vi "ContourPlot multi-channel v1.5.vi"() -> ()   [LabVIEW 2024]
uses:
  <vilib>/Utility/file.llb/Read Delimited Spreadsheet (DBL).vi
  <vilib>/gmath/NI_Gmath.lvlib
  <vilib>/Analysis/NI_AALPro.lvlib
panel:
  out "Channel number":i32=2
  out "Ready?":bool=TRUE
  in  "Tab Control 2":enum32{"Contour"}(tab)
  out "Intensity Graph":dbl[][](graph)
  in  "Begin":i32
  in  "x label index":i32
  in  "y label index":i32=1
  in  "intensisty plot channel index":i32
  in  "y cut x index":i32=1
  in  "length":i32=200
  out "Y cut plot":cluster{dbl[], "Best Polynomial Fit":dbl[]}[](graph)=[{[0.01650390625, 0.02626953125, 0.03503417969, 0.05258789063, 0.06340332031, 0.0546875, 0.07456054687, 0.08317871094, 0.08818359375, 0.09924316406, 0.1127685547, 0.1196777344, 0.1380615234, 0.1424804688, 0.148046875, 0.1650146484, 0.1830322266, 0.1841552734, 0.1907714844, 0.2046386719, 0.2173339844, 0.2219238281, 0.2336425781, 0.2451171875, 0.2626464844, 0.2627197266, 0.2696044922, 0.2876708984, 0.2832763672, 0.2978027344, 0.3136474609, 0.3143798828, 0.3297607422, 0.3401123047, 0.3473144531, 0.355859375, 0.3647460938, 0.3720703125, 0.3781738281, 0.3934082031, 0.4053955078, 0.4169189453, 0.4156494141, 0.4353027344, 0.4502685547, 0.4522949219, 0.4749755859, 0.4762451172, 0.4824707031, 0.4980957031, 0.5044433594, 0.5147216797, 0.5253662109, 0.5385253906, 0.552734375, 0.5608886719, 0.5664306641, 0.5922607422, 0.5865966797, 0.5947509766, 0.6063476562, 0.6142089844, 0.6204345703, 0.6424804687, 0.6439697266, 0.6533691406, 0.6609863281, 0.6897460937, 0.6840820313, 0.7033203125, 0.7142822266, 0.7231201172, 0.7217285156, 0.7270019531, 0.7446777344, 0.7530273438, 0.7546875, 0.7791503906, 0.7783203125, 0.8080810547, 0.8064208984, 0.8069335937, 0.8181640625, 0.8277099609, 0.8401367187, 0.8624023438, 0.8599365234, 0.8799316406, 0.8899169922, 0.8873779297, 0.9, 0.9150390625, 0.9197753906, 0.9276367187, 0.93984375, 0.9463378906, 0.9627929687, 0.9658447266, 0.9845458984, 0.9911865234, 1.010253906, 1.012182617, 1.013989258, 1.03515625, 1.044555664, 1.054956055, 1.057836914, 1.068212891, 1.084838867, 1.094091797, 1.110571289, 1.110839844, 1.119702148, 1.134082031, 1.137158203, 1.161303711, 1.157958984, 1.169970703, 1.183227539, 1.180249023, 1.200537109, 1.208227539, 1.218481445, 1.234399414, 1.243554688, 1.252514648, 1.253100586, 1.276611328, 1.281152344, 1.289453125, 1.303710937, 1.309399414, 1.324316406, 1.327954102, 1.337182617, 1.351611328, 1.34831543, 1.378686523, 1.3796875, 1.387011719, 1.411791992, 1.400170898, 1.414160156, 1.420532227, 1.436669922, 1.440698242, 1.455786133, 1.459790039, 1.479541016, 1.489038086, 1.496142578, 1.511181641, 1.512011719, 1.534008789, 1.534716797, 1.537475586, 1.548364258, 1.570654297, 1.579516602, 1.589624023, 1.589770508, 1.612304687, 1.609423828, 1.624584961, 1.635961914, 1.650219727, 1.652270508, 1.659472656, 1.675244141, 1.690478516, 1.698364258, 1.712353516, 1.714160156, 1.720214844, 1.747485352, 1.749584961, 1.757861328, 1.76862793, 1.776074219, 1.789038086, 1.783422852, 1.798583984, 1.815722656, 1.82565918, 1.828222656, 1.847949219, 1.852368164, 1.857226562, 1.877050781, 1.876049805, 1.894042969, 1.902758789, 1.906469727, 1.93112793, 1.926000977, 1.941088867, 1.946313477, 1.962207031, 1.96887207, 1.978833008], "Best Polynomial Fit"=[2.522949219e-05, 2.175537109e-05, 2.422851563e-05, 2.607177734e-05, 2.364990234e-05, 2.185546875e-05, 2.321044922e-05, 2.395507813e-05, 2.384277344e-05, 2.321289062e-05, 2.442382813e-05, 2.266357422e-05, 2.279052734e-05, 2.379150391e-05, 2.479248047e-05, 2.408935547e-05, 2.789306641e-05, 2.418701172e-05, 2.358154297e-05, 2.761962891e-05, 2.335205078e-05, 2.244384766e-05, 2.471191406e-05, 2.399414063e-05, 2.87890625e-05, 2.490234375e-05, 2.447265625e-05, 2.583496094e-05, 2.252929688e-05, 2.367919922e-05, 2.464111328e-05, 2.297363281e-05, 2.394287109e-05, 2.505371094e-05, 2.201904297e-05, 2.275878906e-05, 2.444824219e-05, 2.458496094e-05, 2.179931641e-05, 2.502685547e-05, 2.063964844e-05, 2.412353516e-05, 2.250976563e-05, 2.124755859e-05, 2.354003906e-05, 2.381835938e-05, 2.278320313e-05, 2.311767578e-05, 2.487548828e-05, 2.473632813e-05, 2.686767578e-05, 2.40234375e-05, 2.554931641e-05, 2.405273438e-05, 2.608398438e-05, 2.446533203e-05, 2.228027344e-05, 2.522705078e-05, 2.221923828e-05, 2.467041016e-05, 2.422851563e-05, 2.247314453e-05, 2.319580078e-05, 2.590332031e-05, 2.395263672e-05, 2.550292969e-05, 2.307617188e-05, 2.522216797e-05, 2.477783203e-05, 2.593261719e-05, 2.587890625e-05, 2.457519531e-05, 2.587646484e-05, 2.187988281e-05, 2.429443359e-05, 2.553222656e-05, 2.353271484e-05, 2.535400391e-05, 2.636474609e-05, 2.397949219e-05, 2.451904297e-05, 2.4453125e-05, 2.314208984e-05, 2.224121094e-05, 2.318847656e-05, 2.693603516e-05, 2.556152344e-05, 2.429443359e-05, 2.602539063e-05, 2.283935547e-05, 2.181640625e-05, 2.506591797e-05, 2.462890625e-05, 2.314941406e-05, 2.465332031e-05, 2.322753906e-05, 2.138671875e-05, 2.248779297e-05, 2.436523437e-05, 2.090576172e-05, 2.705566406e-05, 2.369384766e-05, 2.477783203e-05, 2.453125e-05, 2.129150391e-05, 2.686523438e-05, 2.388671875e-05, 2.263671875e-05, 2.577636719e-05, 2.232421875e-05, 2.777099609e-05, 2.622070313e-05, 2.127441406e-05, 2.596923828e-05, 2.402099609e-05, 2.520263672e-05, 2.533691406e-05, 2.317138672e-05, 2.414550781e-05, 2.462646484e-05, 2.55859375e-05, 2.456054688e-05, 2.296630859e-05, 2.576416016e-05, 2.376220703e-05, 2.401123047e-05, 2.224121094e-05, 2.405029297e-05, 2.700683594e-05, 2.282958984e-05, 2.713867187e-05, 2.715820313e-05, 2.547851562e-05, 2.447265625e-05, 2.329345703e-05, 2.407714844e-05, 1.942382813e-05, 2.3828125e-05, 2.417236328e-05, 2.610107422e-05, 2.278808594e-05, 2.241943359e-05, 2.251220703e-05, 2.4609375e-05, 2.484619141e-05, 2.555908203e-05, 2.657714844e-05, 2.638427734e-05, 2.3515625e-05, 2.619140625e-05, 2.568603516e-05, 2.450683594e-05, 2.463134766e-05, 2.594482422e-05, 2.453125e-05, 2.508056641e-05, 2.398193359e-05, 2.307373047e-05, 2.713867187e-05, 2.829589844e-05, 2.318847656e-05, 2.735839844e-05, 2.381591797e-05, 2.542236328e-05, 2.177001953e-05, 2.354492187e-05, 2.625976563e-05, 2.388427734e-05, 2.348876953e-05, 2.697509766e-05, 2.808837891e-05, 2.255371094e-05, 2.540771484e-05, 2.225097656e-05, 2.594482422e-05, 2.569824219e-05, 2.602539063e-05, 2.532470703e-05, 2.746582031e-05, 2.675537109e-05, 2.2109375e-05, 2.42578125e-05, 2.152587891e-05, 2.559082031e-05, 2.332275391e-05, 2.565917969e-05, 2.493164063e-05, 2.20703125e-05, 2.518798828e-05, 2.071289062e-05, 2.197753906e-05, 2.547851562e-05, 2.424316406e-05, 2.627685547e-05, 2.090576172e-05, 2.405273438e-05, 2.386962891e-05, 2.246826172e-05, 2.632568359e-05, 2.224853516e-05]}, {[0.01650390625, 0.02626953125, 0.03503417969, 0.05258789063, 0.06340332031, 0.0546875, 0.07456054687, 0.08317871094, 0.08818359375, 0.09924316406, 0.1127685547, 0.1196777344, 0.1380615234, 0.1424804688, 0.148046875, 0.1650146484, 0.1830322266, 0.1841552734, 0.1907714844, 0.2046386719, 0.2173339844, 0.2219238281, 0.2336425781, 0.2451171875, 0.2626464844, 0.2627197266, 0.2696044922, 0.2876708984, 0.2832763672, 0.2978027344, 0.3136474609, 0.3143798828, 0.3297607422, 0.3401123047, 0.3473144531, 0.355859375, 0.3647460938, 0.3720703125, 0.3781738281, 0.3934082031, 0.4053955078, 0.4169189453, 0.4156494141, 0.4353027344, 0.4502685547, 0.4522949219, 0.4749755859, 0.4762451172, 0.4824707031, 0.4980957031, 0.5044433594, 0.5147216797, 0.5253662109, 0.5385253906, 0.552734375, 0.5608886719, 0.5664306641, 0.5922607422, 0.5865966797, 0.5947509766, 0.6063476562, 0.6142089844, 0.6204345703, 0.6424804687, 0.6439697266, 0.6533691406, 0.6609863281, 0.6897460937, 0.6840820313, 0.7033203125, 0.7142822266, 0.7231201172, 0.7217285156, 0.7270019531, 0.7446777344, 0.7530273438, 0.7546875, 0.7791503906, 0.7783203125, 0.8080810547, 0.8064208984, 0.8069335937, 0.8181640625, 0.8277099609, 0.8401367187, 0.8624023438, 0.8599365234, 0.8799316406, 0.8899169922, 0.8873779297, 0.9, 0.9150390625, 0.9197753906, 0.9276367187, 0.93984375, 0.9463378906, 0.9627929687, 0.9658447266, 0.9845458984, 0.9911865234, 1.010253906, 1.012182617, 1.013989258, 1.03515625, 1.044555664, 1.054956055, 1.057836914, 1.068212891, 1.084838867, 1.094091797, 1.110571289, 1.110839844, 1.119702148, 1.134082031, 1.137158203, 1.161303711, 1.157958984, 1.169970703, 1.183227539, 1.180249023, 1.200537109, 1.208227539, 1.218481445, 1.234399414, 1.243554688, 1.252514648, 1.253100586, 1.276611328, 1.281152344, 1.289453125, 1.303710937, 1.309399414, 1.324316406, 1.327954102, 1.337182617, 1.351611328, 1.34831543, 1.378686523, 1.3796875, 1.387011719, 1.411791992, 1.400170898, 1.414160156, 1.420532227, 1.436669922, 1.440698242, 1.455786133, 1.459790039, 1.479541016, 1.489038086, 1.496142578, 1.511181641, 1.512011719, 1.534008789, 1.534716797, 1.537475586, 1.548364258, 1.570654297, 1.579516602, 1.589624023, 1.589770508, 1.612304687, 1.609423828, 1.624584961, 1.635961914, 1.650219727, 1.652270508, 1.659472656, 1.675244141, 1.690478516, 1.698364258, 1.712353516, 1.714160156, 1.720214844, 1.747485352, 1.749584961, 1.757861328, 1.76862793, 1.776074219, 1.789038086, 1.783422852, 1.798583984, 1.815722656, 1.82565918, 1.828222656, 1.847949219, 1.852368164, 1.857226562, 1.877050781, 1.876049805, 1.894042969, 1.902758789, 1.906469727, 1.93112793, 1.926000977, 1.941088867, 1.946313477, 1.962207031, 1.96887207, 1.978833008], "Best Polynomial Fit"=[2.3228795830769698e-05, 2.341069346366108e-05, 2.355504147991162e-05, 2.3795519405393273e-05, 2.391469906466257e-05, 2.3820284520124616e-05, 2.401710940979356e-05, 2.4083254900352232e-05, 2.4116888297857293e-05, 2.417975023043444e-05, 2.4237284543491398e-05, 2.4259359660405112e-05, 2.4297365678530806e-05, 2.4302527066994272e-05, 2.430709334103077e-05, 2.4309247635142932e-05, 2.4295677584275923e-05, 2.4294390212520876e-05, 2.4285909030414153e-05, 2.426382232743864e-05, 2.423961165989159e-05, 2.4230148911820358e-05, 2.420474498304174e-05, 2.4178702256432762e-05, 2.413809533096356e-05, 2.413792586502446e-05, 2.4122068153247183e-05, 2.408168103479258e-05, 2.409128550544006e-05, 2.40602426719594e-05, 2.4029119842078877e-05, 2.4027762001171274e-05, 2.4001098745241157e-05, 2.3985289969419927e-05, 2.397537631628508e-05, 2.3964815474921127e-05, 2.3955252565574683e-05, 2.3948480492373423e-05, 2.3943611224214343e-05, 2.3934543789892576e-05, 2.3930494557852824e-05, 2.392912165406224e-05, 2.3929153642764616e-05, 2.393187743218695e-05, 2.393838559748473e-05, 2.3939546312950203e-05, 2.3956771526783283e-05, 2.395795320393103e-05, 2.396405879861498e-05, 2.398151997155728e-05, 2.3989416308291107e-05, 2.4003083872694712e-05, 2.4018271882353802e-05, 2.4038295012871163e-05, 2.4061174823473107e-05, 2.407476876491032e-05, 2.4084159409718046e-05, 2.4128931093897265e-05, 2.41190275799789e-05, 2.413328980614232e-05, 2.4153566159679614e-05, 2.4167231707166706e-05, 2.417796918245362e-05, 2.4215020315544587e-05, 2.421745211179008e-05, 2.423254227494948e-05, 2.4244410577196353e-05, 2.4285688461349103e-05, 2.4278049031381684e-05, 2.4302899628806453e-05, 2.4315592542593103e-05, 2.432499282953925e-05, 2.4323563432301958e-05, 2.432887805523345e-05, 2.4344617917373366e-05, 2.4350907330139375e-05, 2.435206831810665e-05, 2.4365672797342782e-05, 2.4365319581297557e-05, 2.4373213772416386e-05, 2.4373030356769133e-05, 2.4373090207897526e-05, 2.4373686013241878e-05, 2.437313154100677e-05, 2.4370988412561934e-05, 2.436332218384911e-05, 2.436440251089335e-05, 2.4354091150244176e-05, 2.4347690402125148e-05, 2.4349392119753666e-05, 2.434045956135379e-05, 2.4328383364058924e-05, 2.4324291850239552e-05, 2.4317228719890078e-05, 2.4305664413195e-05, 2.4299258201429508e-05, 2.428241499949932e-05, 2.427921642558946e-05, 2.425932582847943e-05, 2.4252212647697625e-05, 2.423196470857647e-05, 2.4229947905135855e-05, 2.4228066279712132e-05, 2.420674559521028e-05, 2.4197845486520096e-05, 2.4188529572252444e-05, 2.4186060654904753e-05, 2.417761630593956e-05, 2.4165736425936328e-05, 2.4160124404331738e-05, 2.4152134496050522e-05, 2.4152027020219336e-05, 2.414891409834052e-05, 2.4145743602599573e-05, 2.4145382808585117e-05, 2.414670574140505e-05, 2.4146067668272524e-05, 2.4149067848212727e-05, 2.4154711883147672e-05, 2.4153226041524322e-05, 2.4165904392509487e-05, 2.4172301617286524e-05, 2.4182216867140978e-05, 2.4200773527796116e-05, 2.4213194961081926e-05, 2.4226583300545907e-05, 2.422750108308381e-05, 2.426854401857523e-05, 2.4277402670570564e-05, 2.429435248766385e-05, 2.432568249131472e-05, 2.4338935906559334e-05, 2.43756213479775e-05, 2.438497239609259e-05, 2.4409364854176795e-05, 2.444929351301051e-05, 2.443999157466549e-05, 2.4529188288595783e-05, 2.453224475064365e-05, 2.455478945062161e-05, 2.463284879451093e-05, 2.459596878044354e-05, 2.4640402371289317e-05, 2.4660763431228958e-05, 2.471233820351259e-05, 2.472515816108467e-05, 2.4772706505834033e-05, 2.478515092076746e-05, 2.4844946786404913e-05, 2.4872482402446116e-05, 2.4892434513846227e-05, 2.4932519173232696e-05, 2.4934637143129816e-05, 2.4986565721917507e-05, 2.4988090871464093e-05, 2.4993939060424103e-05, 2.5015484577399667e-05, 2.50511256715321e-05, 2.5061787335741575e-05, 2.5071280314922957e-05, 2.5071396200998866e-05, 2.508139487184327e-05, 2.508101249043288e-05, 2.5079922617728644e-05, 2.5073917651267062e-05, 2.505981775529839e-05, 2.5057172194115074e-05, 2.5046627692103945e-05, 2.5016614432057417e-05, 2.4978446776763308e-05, 2.495511868258471e-05, 2.4907754575233254e-05, 2.49010838615088e-05, 2.48778136920395e-05, 2.47560482008859e-05, 2.4745568453862603e-05, 2.4702809288685255e-05, 2.4643877542225925e-05, 2.4601077615185943e-05, 2.452297323226292e-05, 2.455733152968015e-05, 2.4462904462535517e-05, 2.4350806303571892e-05, 2.4284071694797085e-05, 2.426672944834396e-05, 2.4132952886881873e-05, 2.41032171235233e-05, 2.4070775940738046e-05, 2.3943019980762065e-05, 2.394922994445811e-05, 2.384325159577108e-05, 2.3797238139455085e-05, 2.3778955372403057e-05, 2.368256158719051e-05, 2.3698512282108175e-05, 2.3658913078691834e-05, 2.365078435756507e-05, 2.3646900161595e-05, 2.365578698321734e-05, 2.3682270055891408e-05]}]
  out "Contour":cluster{dbl[], "Intensity Graph":dbl[]}(graph)={[-1.0, -0.9, -0.8, -0.7, -0.6, -0.5, -0.4, -0.3, -0.2, -0.1, 0.0, 0.1, 0.2, 0.3, 0.4, 0.5, 0.6], "Intensity Graph"=[5100.604889456126, -2470.3463533267786, -634.7944754974578, 10094.369029377345, -5260.545329369828, -207591.59935302305, -1145597.900176921, 501993.89566245984, -411866.74052445486, -492657.58824001026, 1411148.0553569798, 1597.6662420338712, -6432.561102017044, 6389.987173062791, -7753.278633121495, 3521.5036972613993, -2067.527503347544]}
  in  "threshold":dbl=0.18 step=0.01
  in  "extract method":string(combo)="Raw Data"
  in  "book number":i32=786
  in  "file path (dialog if empty)":path=path "C:/Users/gyue/Desktop/20221209 G22L measurement"
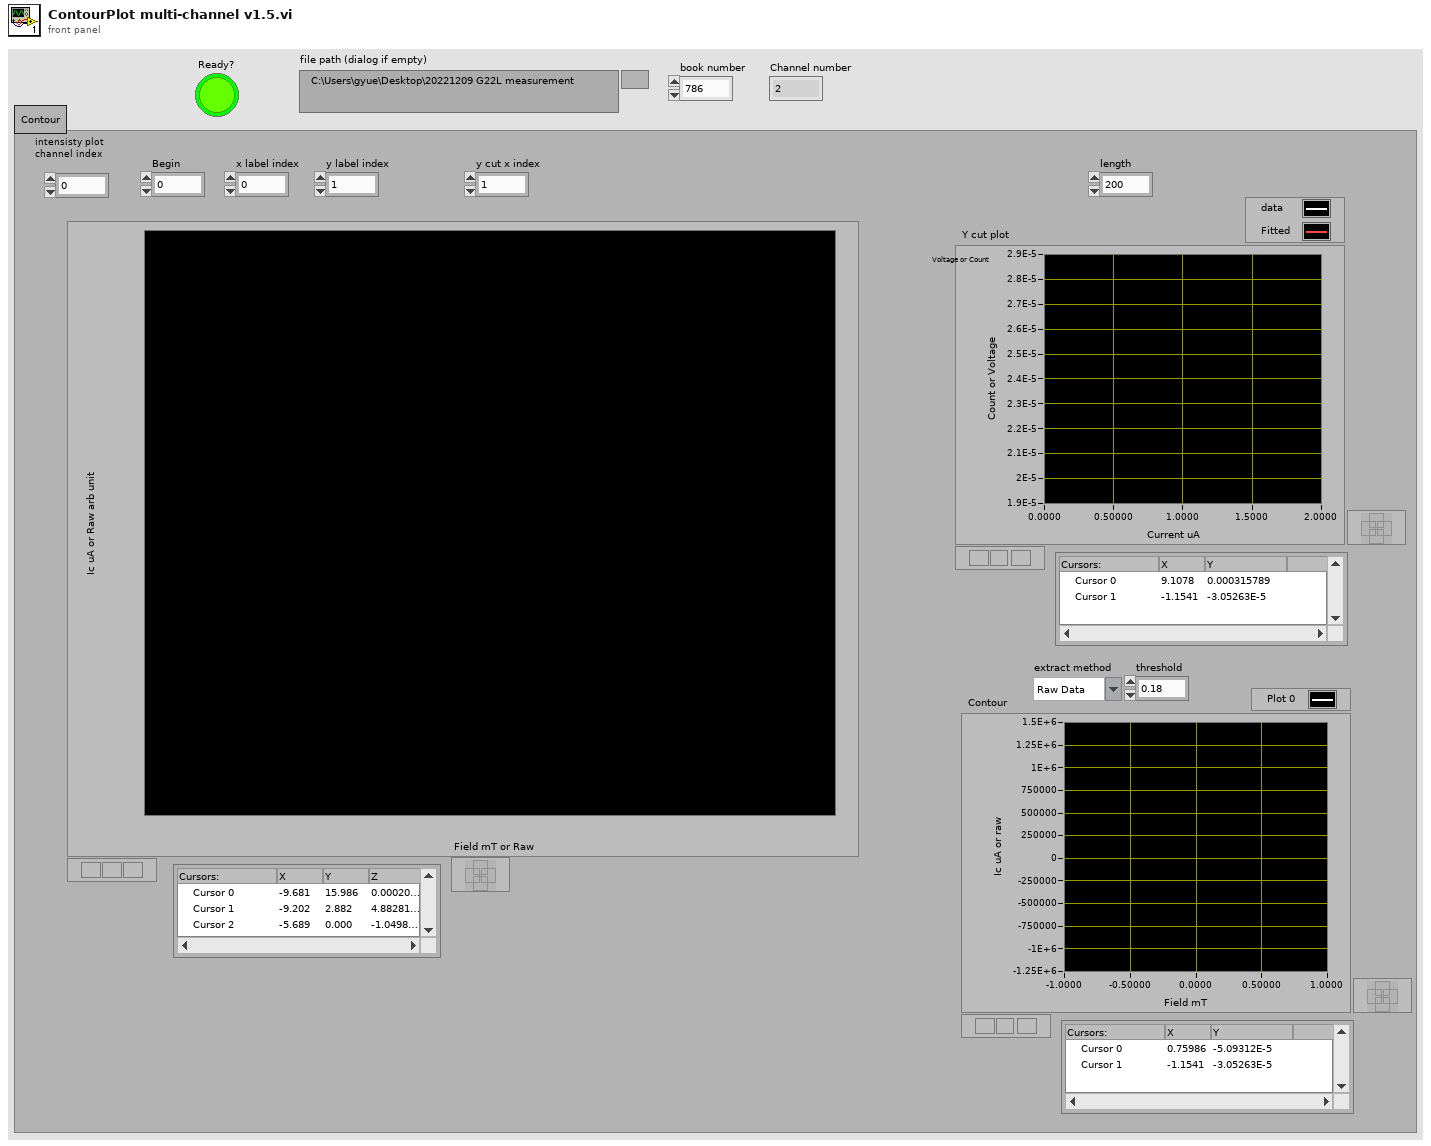
[diagram p1: front panel]
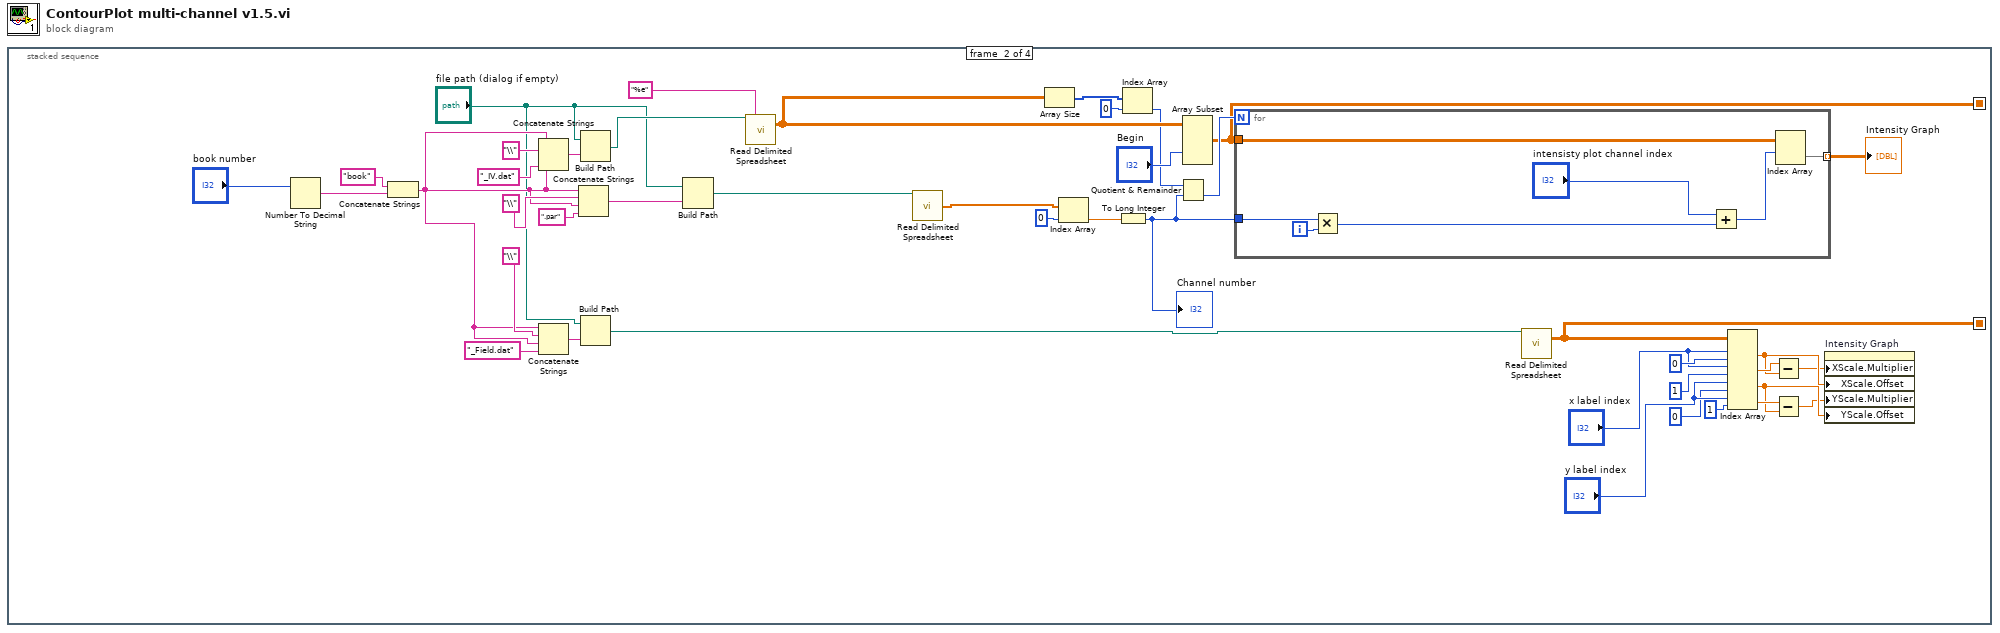
[diagram p0: block diagram]
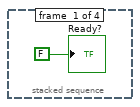
[diagram p2: hidden frame]
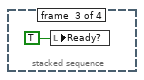
[diagram p3: hidden frame]
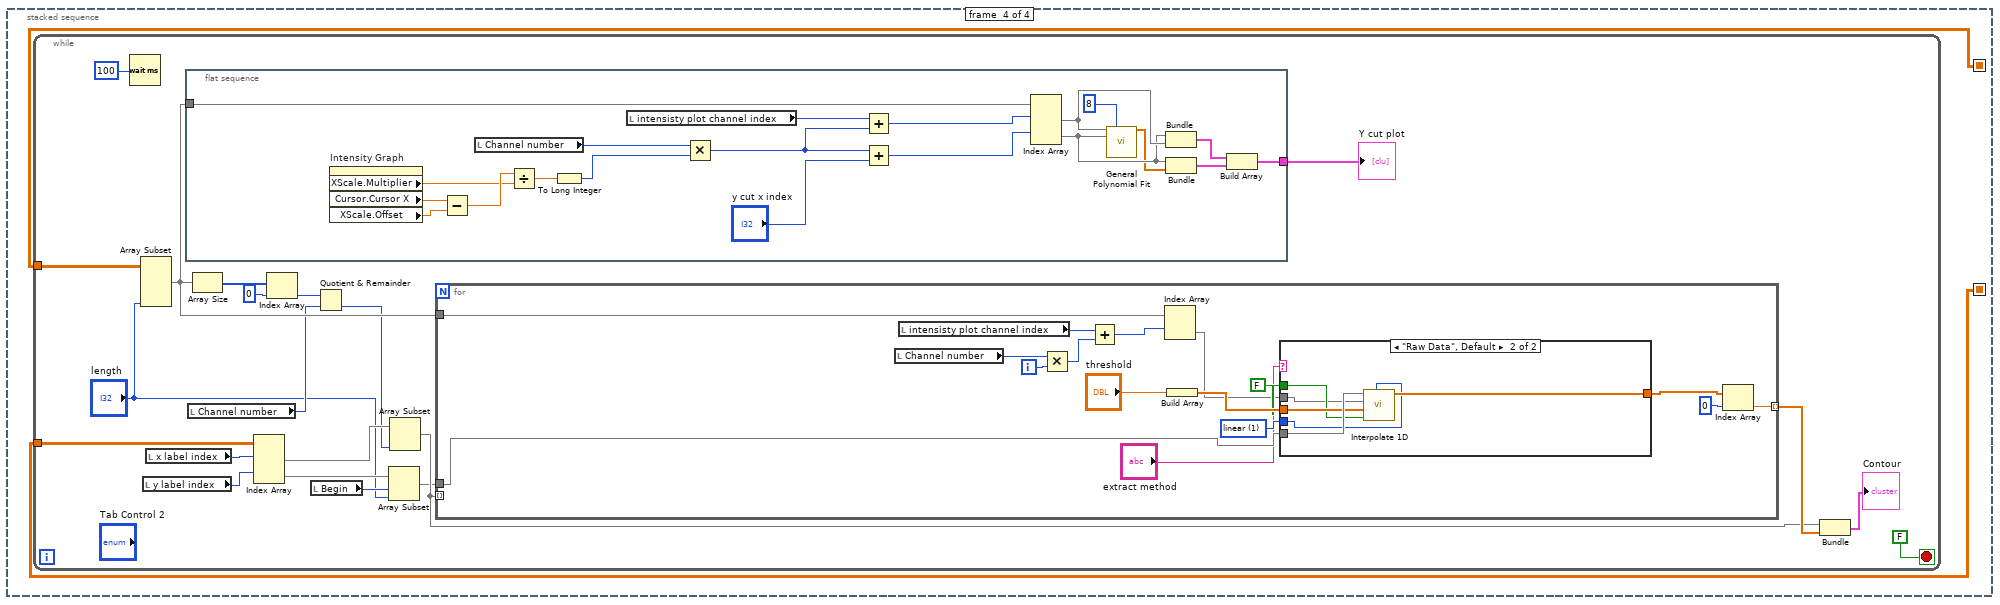
[diagram p4: hidden frame]
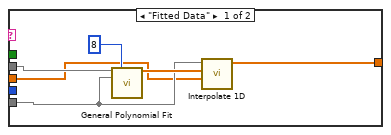
[diagram p5: hidden frame]
diagram:
  n1 = stacked-sequence {
    seq-local: [_ w3 _ _] -> [_ _ _ w53]
    seq-local: [_ w2 _ _] -> [_ _ _ w54]
    frame #0 {
      "Ready?" <- FALSE ("Ready?")
    }
    frame #1 {
      n2 = Number To Decimal String(number="book number") -> (decimal integer string=w40:string)  [unwired: 1 in]
      n3 = Concatenate Strings("book" ("string"), w40) -> (w29:string)
      n4 = Concatenate Strings(w29, "\\" ("string"), w29, "_IV.dat" ("string")) -> (w41:string)
      n5 = Concatenate Strings(w29, "\\" ("string"), w29, "_Field.dat" ("string")) -> (w23:string)
      n6 = Concatenate Strings(w29, "\\" ("string"), w29, ".par" ("string")) -> (w42:string)
      n7 = Build Path(base path="file path (dialog if empty)", name or relative path=w41) -> (appended path=w44:path)
      n8 = Build Path(base path="file path (dialog if empty)", name or relative path=w23) -> (appended path=w16:path)
      n9 = Build Path(base path="file path (dialog if empty)", name or relative path=w42) -> (appended path=w43:path)
      n10 = call-poly <vilib>:"Read Delimited Spreadsheet.vi"("file path (dialog if empty)"=w44, "format (%.3f)"="%e") -> ("all rows"=w26:dbl[][])  [unwired: 8 in, 5 out]
      n11 = call-poly <vilib>:"Read Delimited Spreadsheet.vi"("file path (dialog if empty)"=w43) -> ("first row"=w22:dbl[])  [unwired: 9 in, 5 out]
      n12 = Array Size(array=w26) -> (size(s)=w34:i32[])
      n13 = Index Array(array=w22, index=0) -> (element=w20:dbl)
      n14 = To Long Integer(number=w20) -> (32bit integer=w18:i32)
      "Channel number" <- w18
      n15 = Index Array(array=w34, index=0) -> (element=w19:i32)
      n16 = Quotient & Remainder(x=w19, y=w18) -> (floor(x/y)=w17:i32)  [unwired: 1 out]
      n17 = Array Subset(array=w26, index (col)="Begin") -> (w3:dbl[][])  [unwired: 3 in]
      n18 = for {
        N: w17 -> [_]
        tunnel: w3 -> [w50]
        tunnel: [w49] -> w27 mode=indexing
        tunnel: w18 -> [w46]
        i -> [w51]
        n19 = Multiply(x=w46, y=w51) -> (x*y=w45:i32)
        n20 = Add(x="intensisty plot channel index", y=w45) -> (x+y=w48:i32)
        n21 = Index Array(array=w50, index (row)=w48) -> (element=w49:dbl[])  [unwired: 1 in]
      }
      "Intensity Graph" <- w27
      n22 = call-poly <vilib>:"Read Delimited Spreadsheet.vi"("file path (dialog if empty)"=w16) -> ("all rows"=w2:dbl[][])  [unwired: 9 in, 5 out]
      n23 = Index Array(array=w2, index (row) #1="x label index", index (col) #1=0 ("disabled index (col)"), index (row) #2="x label index", index (col) #2=1 ("disabled index (col)"), index (row) #3="y label index", index (col) #3=0 ("disabled index (col)"), index (row) #4="y label index", index (col) #4=1 ("disabled index (col)")) -> (element #1=w11:dbl, element #2=w12:dbl, element #3=w5:dbl, element #4=w6:dbl)
      n24 = Subtract(x=w12, y=w11) -> (x-y=w10:dbl)
      n25 = Subtract(x=w6, y=w5) -> (x-y=w4:dbl)
      n26 = property on="Intensity Graph" class="IntGraph (strict)"("XScale.Multiplier"=w10, "XScale.Offset"=w11, "YScale.Multiplier"=w4, "YScale.Offset"=w5) -> ()  [unwired: 2 in, 2 out]
    }
    frame #2 {
      n27 = local write "Ready?"(TRUE ("Ready?")) -> ()
    }
    frame #3 {
      n28 = while {
        tunnel: w54 -> [w68]
        tunnel: w53 -> [w67]
        stop <- FALSE stop-if-true
        n29 = Wait (ms)(milliseconds to wait=u32 100) -> ()  [unwired: 1 out]
        n30 = Array Subset(array=w67, length (col)="length") -> (w66:dbl[][])  [unwired: 3 in]
        n31 = local read "y label index"() -> (w70:i32)
        n32 = local read "x label index"() -> (w69:i32)
        n33 = flat-sequence {
          tunnel: [w104] -> w75
          tunnel: w66 -> [w118]
          frame #0 {
            n34 = property on="Intensity Graph" class="IntGraph (strict)"() -> ("XScale.Multiplier"=w122:dbl, "Cursor.Cursor X"=w121:dbl, "XScale.Offset"=w120:dbl)  [unwired: 2 in, 2 out]
            n35 = Subtract(x=w121, y=w120) -> (x-y=w123:dbl)
            n36 = local read "Channel number"() -> (w116:i32)
            n37 = Divide(x=w123, y=w122) -> (x/y=w119:dbl)
            n38 = To Long Integer(number=w119) -> (32bit integer=w117:i32)
            n39 = local read "intensisty plot channel index"() -> (w114:i32)
            n40 = Multiply(x=w116, y=w117) -> (x*y=w115:i32)
            n41 = Add(x=w114, y=w115) -> (x+y=w113:i32)
            n42 = Add(x=w115, y="y cut x index") -> (x+y=w112:i32)
            n43 = Index Array(array=w118, index (row) #1=w113, index (row) #2=w112) -> (element #1=w110:dbl[], element #2=w108:dbl[])  [unwired: 2 in]
            n44 = call <vilib>:"General Polynomial Fit.vi"("Y"=w110, "polynomial order"=8, "X"=w108) -> ("Best Polynomial Fit"=w107:dbl[])  [unwired: 9 in, 3 out]
            n45 = Bundle(w108, w110) -> (w106:cluster{dbl[], dbl[]})  [unwired: 1 in]
            n46 = Bundle(w108, "Best Polynomial Fit"=w107) -> (w105:cluster{dbl[], "Best Polynomial Fit":dbl[]})  [unwired: 1 in]
            n47 = Build Array(w106, w105) -> (w104:cluster{dbl[], "Best Polynomial Fit":dbl[]}[])
          }
        }
        n48 = local read "Channel number"() -> (w62:i32)
        n49 = Array Size(array=w66) -> (size(s)=w65:i32[])
        n50 = Index Array(array=w68, index (row) #1=w69, index (row) #2=w70) -> (element #1=w61:dbl[], element #2=w58:dbl[])  [unwired: 2 in]
        n51 = Index Array(array=w65, index=0) -> (element=w63:i32)
        n52 = local read "Begin"() -> (w57:i32)
        n53 = Quotient & Remainder(x=w63, y=w62) -> (floor(x/y)=w60:i32)  [unwired: 1 out]
        n54 = Array Subset(array=w58, index=w57, length="length") -> (w55:dbl[])
        n55 = Array Subset(array=w61, length=w60) -> (w59:dbl[])  [unwired: 1 in]
        n56 = for {
          tunnel: w66 -> [w91]
          tunnel: w55 -> [w87]
          tunnel: [w88] -> w71 mode=indexing
          tunnel: w59 -> [_] mode=indexing
          i -> [w90]
          w83 = 1 items=["nearest", "linear", "spline", "cubic Hermite", "Lagrange"] ("method")
          n57 = local read "Channel number"() -> (w81:i32)
          n58 = local read "intensisty plot channel index"() -> (w79:i32)
          n59 = Multiply(x=w81, y=w90) -> (x*y=w80:i32)
          n60 = Add(x=w79, y=w80) -> (x+y=w78:i32)
          n61 = Index Array(array=w91, index (row)=w78) -> (element=w77:dbl[])  [unwired: 1 in]
          n62 = Build Array("threshold") -> (w84:dbl[])
          n63 = case shown="\"Raw Data\", Default" "extract method" {
            tunnel: w87 -> [w94 w103]
            tunnel: [w92 w102] -> w86
            tunnel: w84 -> [w93 w101]
            tunnel: w83 -> [_ w100]
            tunnel: FALSE ("X is monotonic") -> [_ w99]
            tunnel: w77 -> [w97 w98]
            frame "Fitted Data" {
              n64 = call <vilib>:"General Polynomial Fit.vi"("Y"=w97, "polynomial order"=8, "X"=w94) -> ("Best Polynomial Fit"=w95:dbl[])  [unwired: 9 in, 3 out]
              n65 = call <vilib>:"Interpolate 1D.vi"("xi"=w93, "X"=w95, "Y"=w94) -> ("yi"=w92:dbl[])  [unwired: 6 in, 2 out]
            }
            frame "Raw Data", Default {
              n66 = call <vilib>:"Interpolate 1D.vi"("method"=w100, "X is monotonic"=w99, "xi"=w101, "X"=w98, "Y"=w103) -> ("yi"=w102:dbl[])  [unwired: 4 in, 2 out]
            }
          }
          n67 = Index Array(array=w86, index=0) -> (element=w88:dbl)
        }
        n68 = Bundle(w59, w71) -> (→"Contour":cluster{dbl[], dbl[]})  [unwired: 1 in]
        "Y cut plot" <- w75
      }
    }
  }
